vi "Offsets Widget.vi"(8 "error in (no error)":errorcluster) -> (0 "error out":errorcluster)   [LabVIEW 2013]
uses:
  Popups/Update Offset Actions.ctl
  lib/Data Access Objects/Metadata/Persistant DAO Actions.ctl
  lib/Data Access Objects/Metadata/DAO Actions.ctl
  lib/Global Data/Transactions/Dataset Source.ctl
  lib/Global Data/Transactions/Dataset Type.ctl
  lib/Apps/Yes No Button.ctl
  lib/Global Data/Transactions/Dataset Transaction Id.ctl
  lib/Data Access Objects/Metadata/DAO Actions with Remove.ctl
  lib/Launcher/Launcher Actions.ctl
  lib/Launcher/NoPanelAppTypes.ctl
  lib/Offsets/Offset Types.ctl
  Popups/Offset Message.ctl
  <vilib>/Utility/miscctls.llb/LVPointTypeDef.ctl
  lib/Data Display/External Sensor Name Offset & Value.ctl
  lib/Offsets Widget/Offset Widget Actions.ctl
  lib/MixedMode/Messages/MM Widget Parameter Changes.ctl
  lib/Apps/GUI Control.ctl
  lib/Data Access Objects/Sensors/Sensor List Class.lvclass
  Popups/Offset Table Component.ctl
  lib/Offsets Widget/Cartesian Or Actuator.ctl
panel:
  in  "HasBeenModified":bool
  in  "External Sensors Label":string[](array[string])
  in  "External Sensors Table":T1[](array[typedef])
  in  "Table 5":T2 {"Table Data 1" format="%^#_7e"}
  in  "Table 4":T2 {"Table Data 1" format="%^#_7e"}
  in  "Table 3":T2 {"Table Data 1" format="%^#_7e"}
  in  "Table 2":T2 {"Table Data 1" format="%^#_7e"}
  in  "Table 1":T2 {"Table Data 1" format="%^#_7e"}
  in  "Row Labels":string[](array[string])
  in  "Table 0":T2 {"Table Data 1" format="%^#_7e"}
  out "Default Data":dbl[][](array[numeric])
  out "Default Transactions":T3[](array[typedef])
  in  "Coordinate Space":T7 caption="Coord"
  in  "Cartesian Type":bool caption="Coord"
  in  "Offset Type":T8
  in  "Load":bool
  in  "Number Of Samples":i32
  in  "Sample Interval\n(milliseconds)":dbl
  in  "Offset Widget Actions":T9
  in  "Execute":bool
  in  "Cancel":bool
  in  "Ok":bool
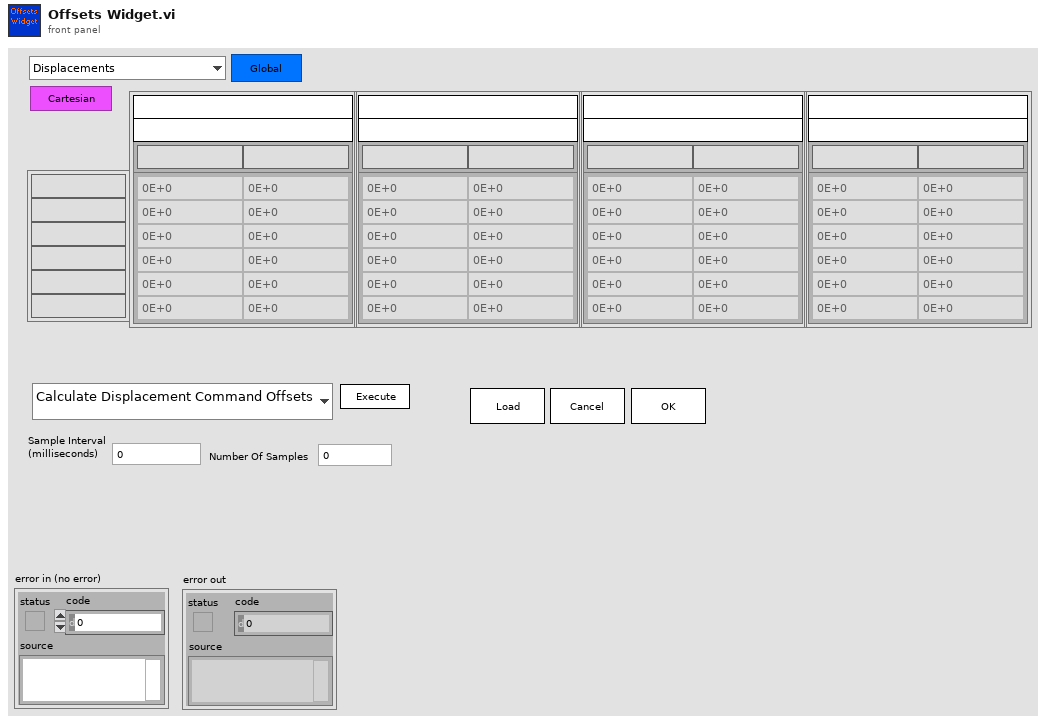
[diagram p1: front panel]
types:
  T1 = typedef "External Sensor Name Offset & Value.ctl" = cluster{"Name":string, "Offset":dbl, "Value 2":dbl}
  T2 = typedef "Offset Table Component.ctl" = cluster{"Table Data 1":dbl[][], "Offset or Current Label":string[], "DOF Label":string, "LBCB Label":string}
  T3 = typedef "Dataset Transaction Id.ctl" = cluster{"Dataset Source":T4, "Dataset Type":T5, "Hold":T6, "Volts":T6, "Tag":string}
  T4 = typedef "Dataset Source.ctl" = enum16{"Continuous", "Hold", "ED", "Volts", "Offsets", "Increments"}
  T5 = typedef "Dataset Type.ctl" = enum16{"LVDT", "Load Cell", "Actuator Command", "Servo Error", "Displacement Command", "Displacement", "Force"}
  T6 = typedef "Yes No Button.ctl" = bool
  T7 = typedef "Cartesian Or Actuator.ctl" = bool
  T8 = typedef "Offset Types.ctl" = enum16{"Displacements", "Forces", "External Sensors"}
  T9 = typedef "Offset Widget Actions.ctl" = enum16{"Calculate Displacement Command Offsets", "Calculate Displacement Offsets", "Calculate Force Offsets", "Calculate External Sensor Offsets"}
  T10 = typedef "GUI Control.ctl" = cluster{"Command":T11, "LBCB Number":enum16{"LBCB1", "LBCB2"}}
  T11 = typedef "MM Widget Parameter Changes.ctl" = enum16{"Start", "Stop All", "Control Enabled", "Control Disabled"}
  T12 = typedef "Offset Message.ctl" = cluster{"Update Offset Actions":T13, "Offset Type":T8, "Coordinate Space":bool, "Cartesian Type":bool}
  T13 = typedef "Update Offset Actions.ctl" = enum16{"Update Table", "Calculate Cartesian Offsets", "Redo Headers", "Has Been Modified", "Exit"}
  T14 = typedef "LVPointTypeDef.ctl" = cluster{"Horizontal":i16, "Vertical":i16}
  T15 = typedef "Persistant DAO Actions.ctl" = enum16{"Init", "Get", "Set", "Load", "Save"}
  T16 = typedef "DAO Actions.ctl" = enum16{"Init", "Get", "Set"}
  T17 = typedef "LVRectTypeDef.ctl" = cluster{"Left":i16, "Top":i16, "Right":i16, "Bottom":i16}
  T18 = typedef "App Parameters.ctl" = cluster{"Monitor Loop":T19, "Ramp Time":T19, "Log Loop":T19, "TCP to DAQ":T19, "Logging Directory":path, "Log File Size (MBytes)":i64, "Volt Logging Loop":T19, "2 LBCB Archiving Mode":bool, "Fake":bool}
  T19 = typedef "Timing Parameters.ctl" = cluster{"Interval":dbl, "Rate ":dbl}
  T20 = typedef "Number Of LBCBs.ctl" = enum16{"1", "2"}
  T21 = cluster{"Table Data 1":dbl[][], "Offset or Current Label":string[], "DOF Label":string, "LBCB Label":string}
  T22 = typedef "DAO Actions with Remove.ctl" = enum16{"Init", "Get", "Set", "Remove"}
  T23 = typedef "NoPanelAppTypes.ctl" = enum16{"NTCP Socket", "Data Archiving", "DAQ Link", "Control Loops", "Cmd Disp Diffs", "LBCB Data", "Limits", "Mixed Mode Widget", "Offsets", "Debug"}
  T24 = typedef "Launcher Actions.ctl" = enum16{"Launch", "Stop All", "Stop", "Kill", "Running?", "Init"}
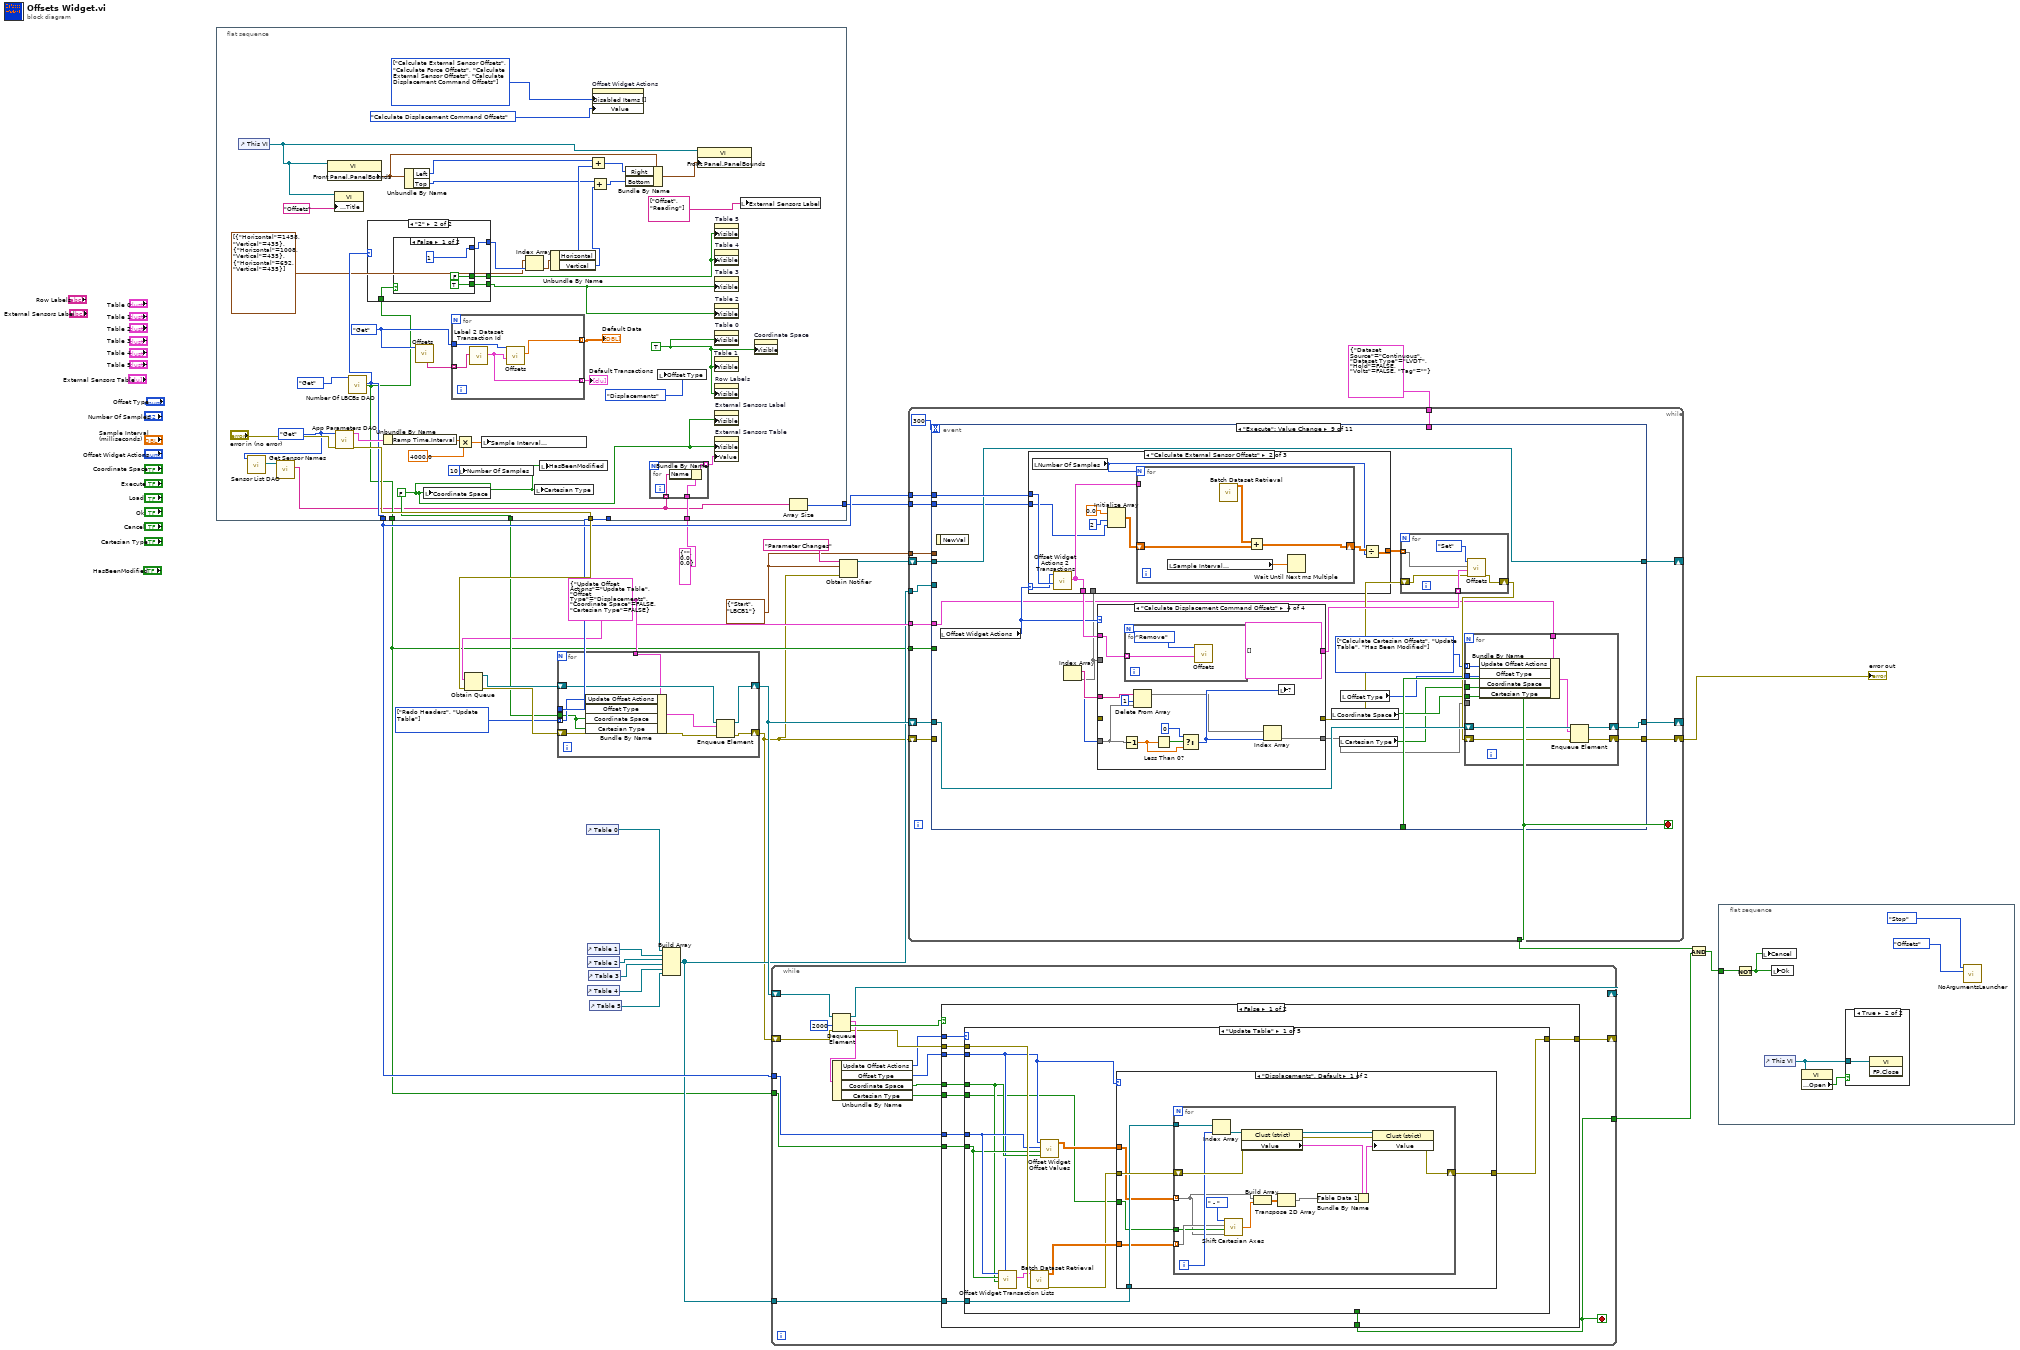
[diagram p0: block diagram]
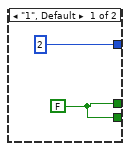
[diagram p2: hidden frame]
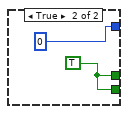
[diagram p3: hidden frame]
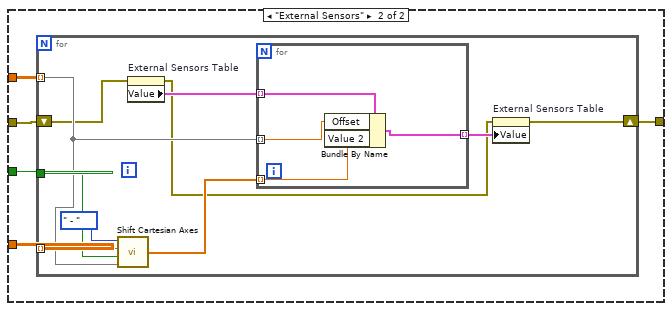
[diagram p5: hidden frame]
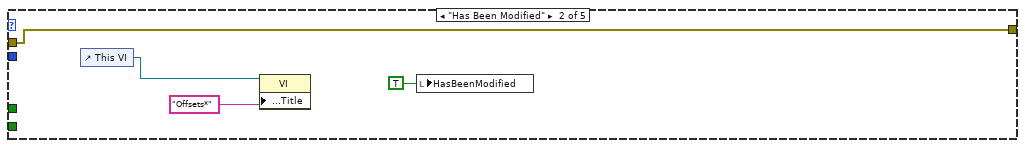
[diagram p6: hidden frame]
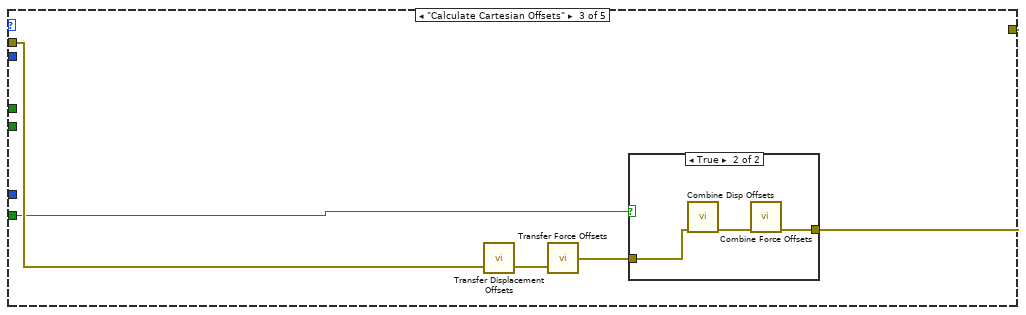
[diagram p7: hidden frame]
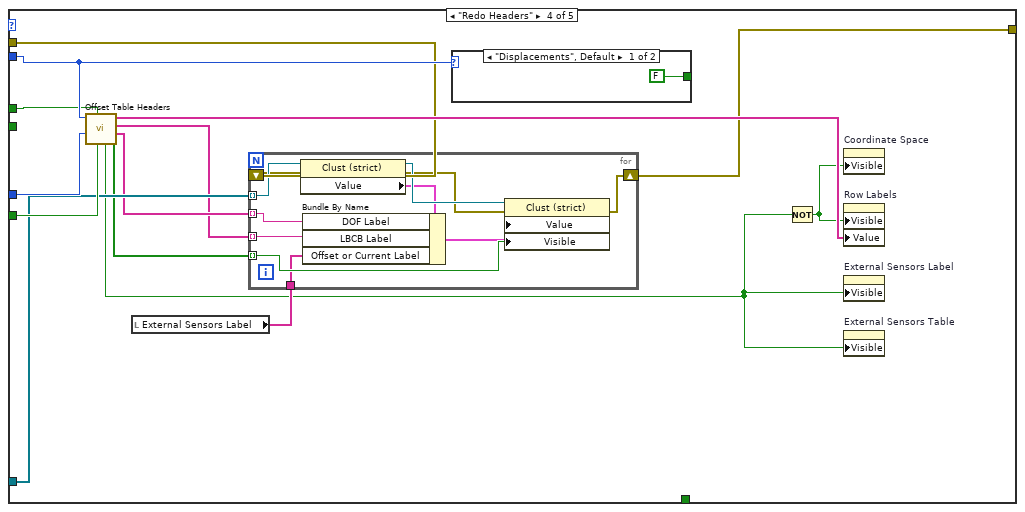
[diagram p9: hidden frame]
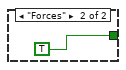
[diagram p10: hidden frame]
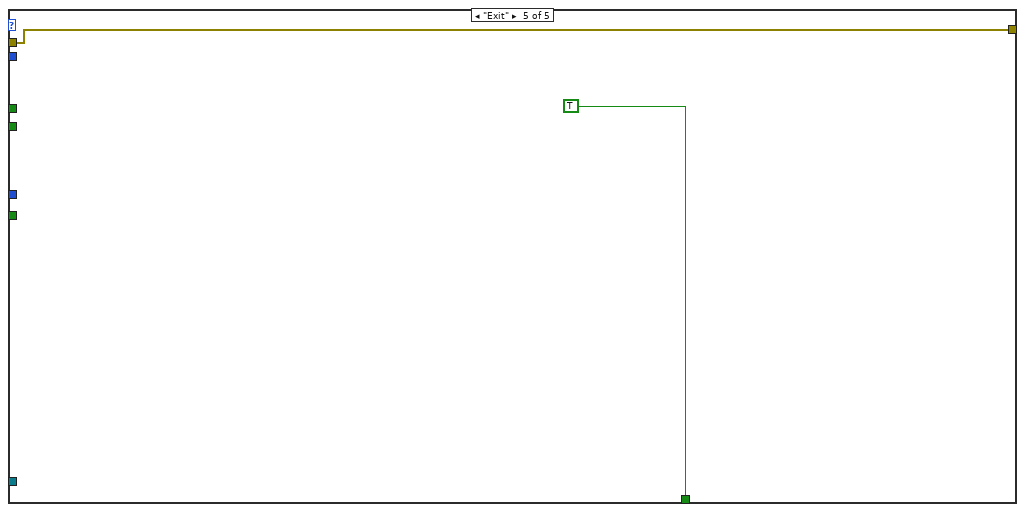
[diagram p11: hidden frame]
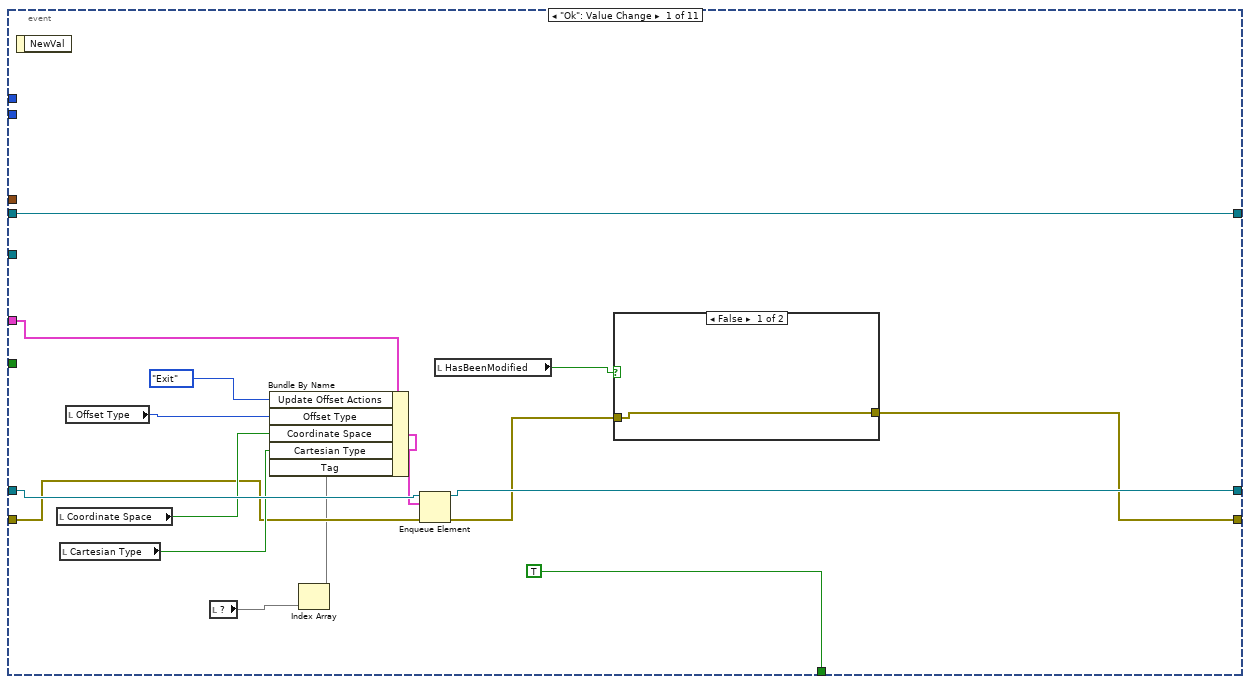
[diagram p13: hidden frame]
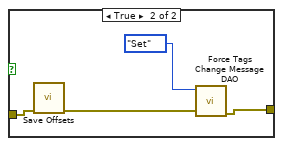
[diagram p14: hidden frame]
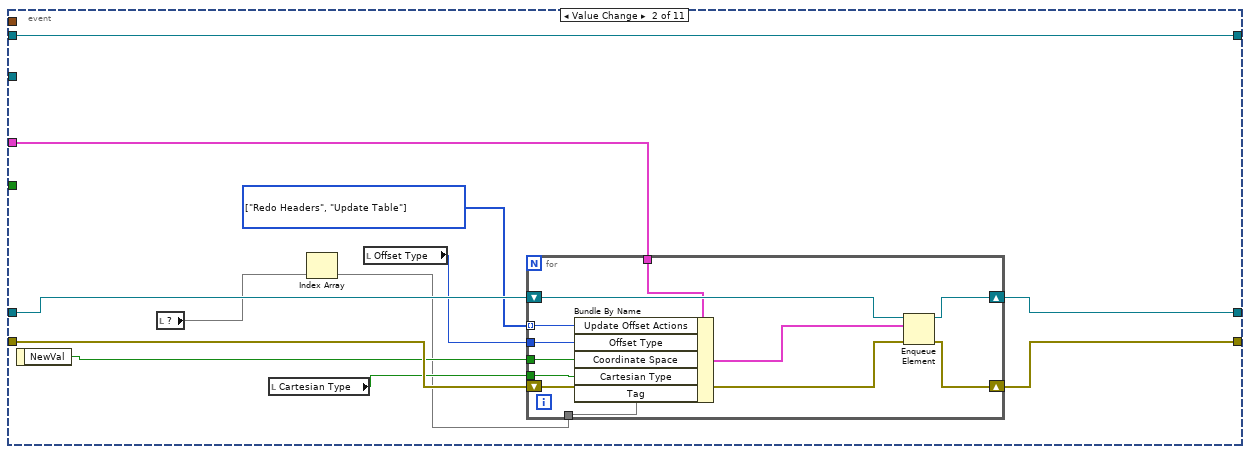
[diagram p15: hidden frame]
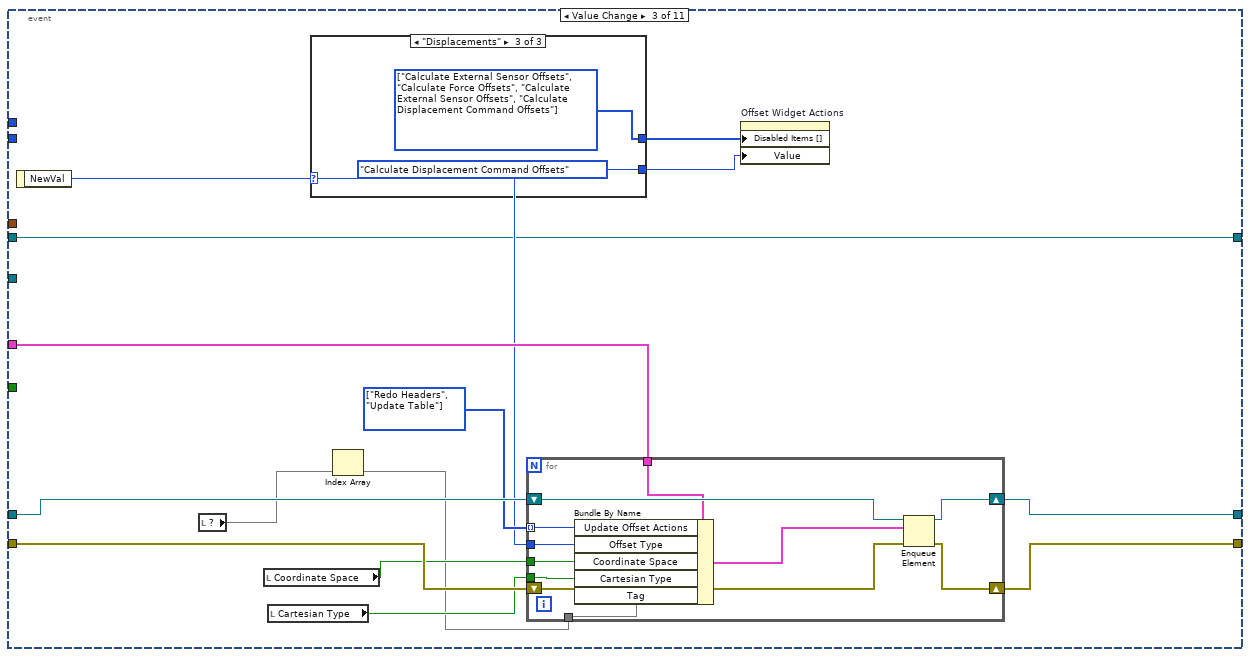
[diagram p16: hidden frame]
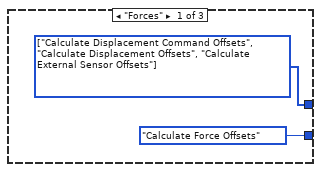
[diagram p17: hidden frame]
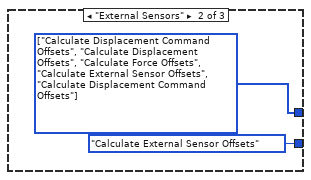
[diagram p18: hidden frame]
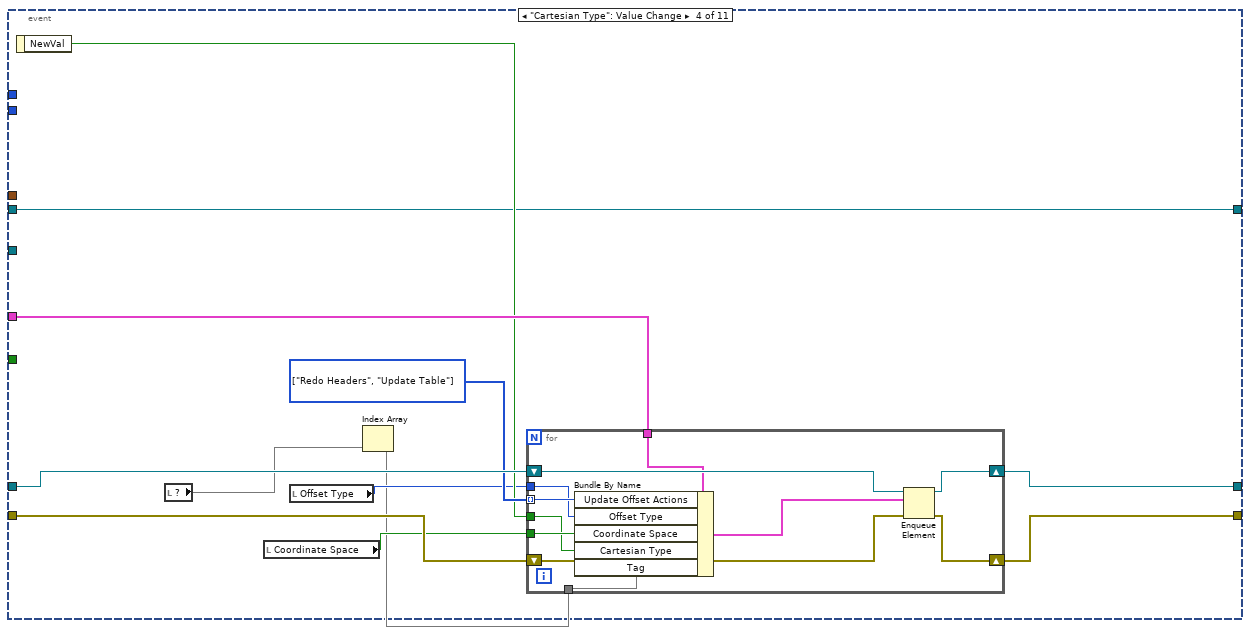
[diagram p19: hidden frame]
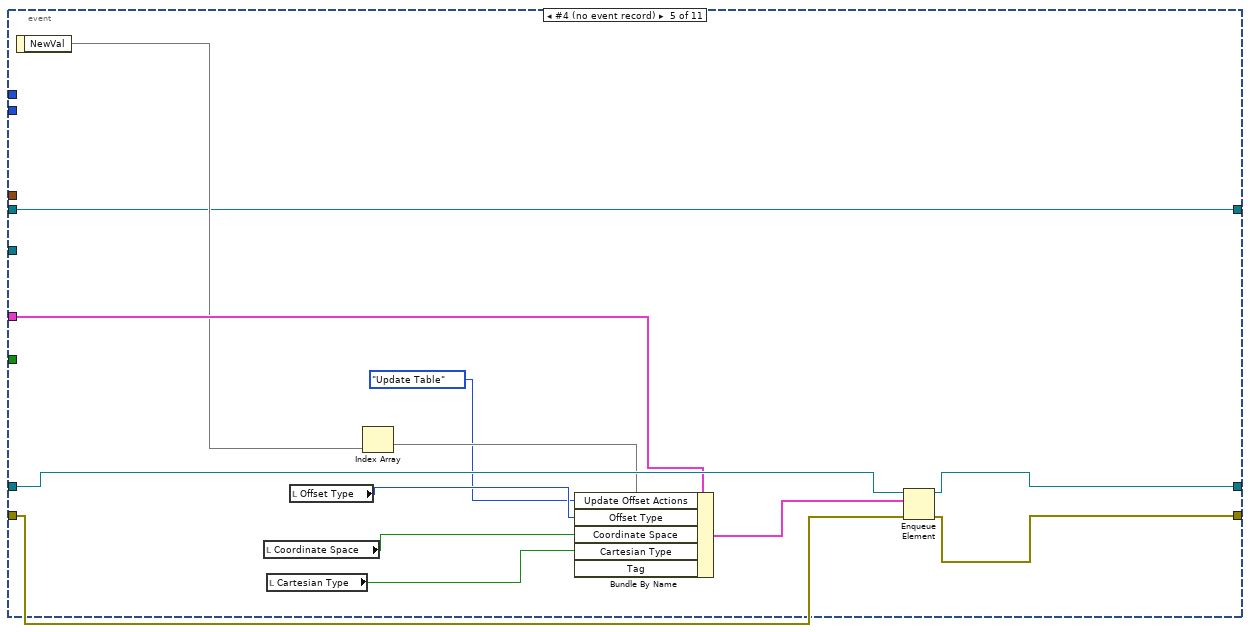
[diagram p20: hidden frame]
diagram:
  w2 = T10 {"Command"=enum."Start", "LBCB Number"=enum."LBCB1"} ("GUI Control")
  w16 = T12 {"Update Offset Actions"=enum."Update Table", "Offset Type"=enum."Displacements", "Coordinate Space"=FALSE, "Cartesian Type"=FALSE} ("Offset Message")
  w19 = T13[] [enum."Redo Headers", enum."Update Table"] items=["Update Table", "Calculate Cartesian Offsets", "Redo Headers", "Has Been Modified", "Exit"]
  n1 = flat-sequence {
    tunnel: [w59] -> w21
    tunnel: [w57] -> w20
    tunnel: [w56] -> w6
    tunnel: [w29] -> w18
    tunnel: [w35] -> w17
    tunnel: T1 {"Name"="", "Offset"=0.0, "Value 2"=0.0} ("External Sensor Name & Value") -> [w49]
    tunnel: [w33] -> w1
    frame #0 {
      w39 = T9[] [enum."Calculate External Sensor Offsets", enum."Calculate Force Offsets", enum."Calculate External Sensor Offsets", enum."Calculate Displacement Command Offsets"] items=["Calculate Displacement Command Offsets", "Calculate Displacement Offsets", "Calculate Force Offsets", "Calculate External Sensor Offsets"] ("Disabled Items []")
      w34 = TRUE ("Visible")
      w35 = FALSE ("Coordinate Space")
      w60 = DAO_Actions."Get" ("DAO Actions")
      w31 = Persistant_DAO_Actions."Get" ("Actions")
      n2 = control-ref of="This VI"() -> (w37:refnum<vi>)
      n3 = call "Sensor List DAO.vi"("Actions"=w31) -> ("Sensor List Out"=w32:refnum<class "Sensor List Class.lvclass">)  [unwired: 8 in, 2 out]
      n4 = call "Get Sensor Names.vi"("Sensor List Class in"=w32) -> ("Names"=w30:string[])  [unwired: 8 in, 2 out]
      n5 = property class="VI"(reference=w37) -> ("Front Panel.PanelBounds"=w44:T17)  [unwired: 1 in, 2 out]
      n6 = property class="VI"(reference=w37, "Front Panel.Title"="Offsets" ("Front Panel Window:Title")) -> ()  [unwired: 1 in, 2 out]
      n7 = call "App Parameters DAO.vi"("error in (no error)"="error in (no error)", "Actions"=w31) -> ("error out"=w59:errorcluster, "Application Timing and Logging Out"=w66:T18)  [unwired: 2 in, 6 out]
      n8 = call "Number Of LBCBs DAO.vi"("Actions"=Persistant_DAO_Actions."Get") -> ("Number of\nLBCBs Out"=w57:T20, "Rigid Connection Out"=w56:bool)  [unwired: 13 in, 4 out]
      n9 = case shown="\"2\"" w57 {
        tunnel: w56 -> [_ w79]
        tunnel: [2 w78] -> w55
        tunnel: [w74 w77] -> w52
        tunnel: [w74 w76] -> w51
        frame "1", Default {
          w74 = FALSE
        }
        frame "2" {
          n10 = case shown="False" w79 {
            tunnel: [1 ("f") 0] -> w78
            tunnel: [FALSE w83] -> w77
            tunnel: [TRUE w83] -> w76
            frame False {
            }
            frame True {
              w83 = TRUE
            }
          }
        }
      }
      n11 = Unbundle By Name(w66) -> ("Ramp Time.Interval"=w67:dbl)
      n12 = Unbundle By Name(w44) -> ("Left"=w48:i16, "Top"=w46:i16)
      n13 = call "Offsets.vi"("DAO Actions"=w60) -> ("Labels"=w64:string[])  [unwired: 8 in, 2 out]
      n14 = local write "Coordinate Space"(w35) -> ()
      n15 = for {
        tunnel: w64 -> [w88] mode=indexing
        tunnel: w60 -> [w87]
        tunnel: [w86] -> w63 mode=indexing
        tunnel: [w85] -> w62 mode=indexing
        n16 = call "Label 2 Dataset Transaction Id.vi"("Label"=w88) -> ("Dataset Trans Id"=w86:T3)  [unwired: 10 in]
        n17 = call "Offsets.vi"("Dataset Trans Id"=w86, "DAO Actions"=w87) -> ("Data Out"=w85:dbl[])  [unwired: 7 in, 2 out]
      }
      "Default Transactions" <- w63
      "Default Data" <- w62
      n18 = Multiply(x=w67, y=4000.0) -> (x*y=w69:dbl)
      n19 = local write "Number Of Samples"(10 ("Number Of Samples")) -> ()
      n20 = local write "Sample Interval\n(milliseconds)"(w69) -> ()
      n21 = Index Array(array=T14[] [{"Horizontal"=1458, "Vertical"=435}, {"Horizontal"=1008, "Vertical"=435}, {"Horizontal"=692, "Vertical"=435}], index=w55) -> (element=w53:T14)
      n22 = local write "Cartesian Type"(w35) -> ()
      n23 = local write "HasBeenModified"(w35) -> ()
      n24 = Unbundle By Name(w53) -> ("Horizontal"=w47:i16, "Vertical"=w45:i16)
      n25 = Add(x=w48, y=w47) -> (x+y=w42:i16)
      n26 = Add(x=w46, y=w45) -> (x+y=w41:i16)
      n27 = property on="Offset Widget Actions" class="Enum (strict)"("Disabled Items []"=w39, "Value"=Offset_Widget_Actions."Calculate Displacement Command Offsets" ("Offset Widget Actions")) -> ()  [unwired: 2 in, 2 out]
      n28 = Bundle By Name(cluster=w44, "Right"=w42, "Bottom"=w41) -> (w43:T17)
      n29 = for {
        tunnel: [w73] -> w50 mode=indexing
        tunnel: w49 -> [w72]
        tunnel: w30 -> [w71] mode=indexing
        n30 = Bundle By Name(cluster=w72, "Name"=w71) -> (w73:T1)
      }
      n31 = local write "Offset Type"(Offset_Types."Displacements" ("Offset Type")) -> ()
      n32 = property class="VI"(reference=w37, "Front Panel.PanelBounds"=w43) -> ()  [unwired: 1 in, 2 out]
      n33 = property on="Table 5" class="Clust (strict)"("Visible"=w52) -> ()  [unwired: 2 in, 2 out]
      n34 = property on="Table 4" class="Clust (strict)"("Visible"=w52) -> ()  [unwired: 2 in, 2 out]
      n35 = property on="Table 3" class="Clust (strict)"("Visible"=w51) -> ()  [unwired: 2 in, 2 out]
      n36 = property on="Table 2" class="Clust (strict)"("Visible"=w51) -> ()  [unwired: 2 in, 2 out]
      n37 = property on="Table 0" class="Clust (strict)"("Visible"=w34) -> ()  [unwired: 2 in, 2 out]
      n38 = property on="Table 1" class="Clust (strict)"("Visible"=w34) -> ()  [unwired: 2 in, 2 out]
      n39 = property on="Row Labels" class="Arr (strict)"("Visible"=w34) -> ()  [unwired: 2 in, 2 out]
      n40 = property on="External Sensors Label" class="Arr (strict)"("Visible"=w35) -> ()  [unwired: 2 in, 2 out]
      n41 = property on="External Sensors Table" class="Arr (strict)"("Visible"=w35, "Value"=w50) -> ()  [unwired: 2 in, 2 out]
      n42 = local write "External Sensors Label"(string[] ["Offset", "Reading"] ("External Sensors Label")) -> ()
      n43 = property on="Coordinate Space" class="Bool (strict)"("Visible"=w34) -> ()  [unwired: 2 in, 2 out]
      n44 = Array Size(array=w30) -> (size(s)=w33:i32)
    }
  }
  n45 = Obtain Queue(element data type=w16, error in (no error)=w21) -> (queue out=w27:refnum<queue>, error out=w28:errorcluster)  [unwired: 3 in, 1 out]
  n46 = for {
    tunnel: w19 -> [w93] mode=indexing
    shift-right: [w94] -> w26
    shift-left: w27 -> [w95]
    shift-right: [w92] -> w3
    shift-left: w28 -> [w96]
    tunnel: w16 -> [w90]
    tunnel: w18 -> [_]
    tunnel: w17 -> [w89]
    n47 = Bundle By Name(cluster=w90, "Update Offset Actions"=w93, "Coordinate Space"=w89, "Cartesian Type"=w89) -> (w91:T12)  [unwired: 1 in]
    n48 = Enqueue Element(queue=w95, element=w91, error in (no error)=w96) -> (queue out=w94:refnum<queue>, error out=w92:errorcluster)  [unwired: 1 in, 1 out]
  }
  n49 = control-ref of="Table 0"() -> (w15:refnum<vi>)
  n50 = control-ref of="Table 1"() -> (w14:refnum<vi>)
  n51 = control-ref of="Table 2"() -> (w13:refnum<vi>)
  n52 = control-ref of="Table 4"() -> (w11:refnum<vi>)
  n53 = control-ref of="Table 3"() -> (w12:refnum<vi>)
  n54 = control-ref of="Table 5"() -> (w10:refnum<vi>)
  n55 = Build Array(w15, w14, w13, w12, w11, w10) -> (w8:refnum<vi>[])
  n56 = while {
    shift-right: [w109] -> _
    shift-left: w26 -> [w111]
    shift-right: [w105] -> _
    shift-left: w3 -> [w110]
    tunnel: [w104] -> w23
    tunnel: w20 -> [w103]
    tunnel: w6 -> [w102]
    tunnel: w8 -> [w98]
    stop <- w104 stop-if-true
    n57 = Dequeue Element(queue=w111, timeout in ms (-1)=2000, error in (no error)=w110) -> (queue out=w109:refnum<queue>, element=w107:T12, timed out?=w108:bool, error out=w106:errorcluster)
    n58 = Unbundle By Name(w107) -> ("Update Offset Actions"=w101:T13, "Offset Type"=w100:T8, "Coordinate Space"=w99:bool, "Cartesian Type"=w97:bool)
    n59 = case shown="False" w108 {
      tunnel: w101 -> [w122 _]
      tunnel: w106 -> [w121 w219]
      tunnel: [w120 w219] -> w105
      tunnel: [w119 _] -> w104
      tunnel: w100 -> [w118 _]
      tunnel: w103 -> [w117 _]
      tunnel: w102 -> [w116 _]
      tunnel: w99 -> [w115 _]
      tunnel: w98 -> [w114 _]
      tunnel: w97 -> [w113 _]
      frame False {
        n60 = case shown="\"Update Table\"" w122 {
          tunnel: w121 -> [w134 w176 w181 w192 w217]
          tunnel: [w125 w176 w183 w193 w217] -> w120
          tunnel: [_ _ _ _ TRUE] -> w119
          tunnel: w118 -> [w124 _ _ w202 _]
          tunnel: w117 -> [w131 _ _ w201 _]
          tunnel: w116 -> [w130 _ w180 w199 _]
          tunnel: w115 -> [w129 _ _ w200 _]
          tunnel: w114 -> [w127 _ _ w197 _]
          tunnel: w113 -> [w123 _ _ _ _]
          frame "Update Table" {
            n61 = call "Offset Widget Transaction Lists.vi"("Offset Type"=w124, "Coordinate Space"=w129, "Rigid Connection"=w130, "Number of\nLBCBs"=w131) -> ("Transactions"=w128:T3[])  [unwired: 6 in, 1 out]
            n62 = call "Batch Dataset Retrieval.vi"("error in"=w134, "Transactions"=w128) -> ("error out"=w126:errorcluster, "Data"=w133:dbl[][])  [unwired: 8 in]
            n63 = call "Offset Widget Offset Values.vi"("Coordinate Space"=w129, "Rigid Connection In"=w130, "Number of\nLBCBs"=w131, "Offset Type"=w124) -> ("Offsets"=w132:dbl[][])  [unwired: 7 in]
            n64 = case shown="\"Displacements\", Default" w124 {
              tunnel: w133 -> [w137 w161]
              tunnel: w132 -> [w136 w160]
              tunnel: w123 -> [w135 w159]
              tunnel: w127 -> [w138 _]
              tunnel: w126 -> [w140 w158]
              tunnel: [w139 w157] -> w125
              frame "Displacements", Default {
                n65 = for {
                  shift-right: [w154] -> w139
                  shift-left: w140 -> [w156]
                  tunnel: w138 -> [w153]
                  tunnel: w137 -> [w147] mode=indexing
                  tunnel: w136 -> [w145] mode=indexing
                  tunnel: w135 -> [w146]
                  i -> [w152]
                  n66 = Index Array(array=w153, index=w152) -> (element=w151:refnum<vi>)
                  n67 = call "Shift Cartesian Axes.vi"("Coordinate Offset"=w145, "Coordinate Switch"=w146, "Coordinate Input"=w147, "Direction"=enum16{" +", " - "}." - ") -> ("Coordinate Output"=w144:dbl[])
                  n68 = property class="Clust (strict)"(reference=w151, error in=w156) -> (reference out=w150:refnum<vi>, error out=w155:errorcluster, "Value"=w149:T21)
                  n69 = Build Array(w145, w144) -> (w143:dbl[][])
                  n70 = Transpose 2D Array(2D array=w143) -> (transposed array=w142:dbl[][])
                  n71 = Bundle By Name(cluster=w149, "Table Data 1"=w142) -> (w141:T21)
                  n72 = property class="Clust (strict)"(reference=w150, error in=w155, "Value"=w141) -> (error out=w154:errorcluster)  [unwired: 1 out]
                }
              }
              frame "External Sensors" {
                n73 = for {
                  tunnel: w161 -> [w171] mode=indexing
                  tunnel: w159 -> [w170]
                  tunnel: w160 -> [w167] mode=indexing
                  shift-right: [w164] -> w157
                  shift-left: w158 -> [w163]
                  n74 = call "Shift Cartesian Axes.vi"("Coordinate Offset"=w167, "Coordinate Switch"=w170, "Coordinate Input"=w171, "Direction"=enum16{" +", " - "}." - ") -> ("Coordinate Output"=w166:dbl[])
                  n75 = property on="External Sensors Table" class="Arr (strict)"(error in=w163) -> (error out=w162:errorcluster, "Value"=w168:T1[])  [unwired: 1 in, 1 out]
                  n76 = for {
                    tunnel: w168 -> [w175] mode=indexing
                    tunnel: w167 -> [w174] mode=indexing
                    tunnel: w166 -> [w173] mode=indexing
                    tunnel: [w172] -> w165 mode=indexing
                    n77 = Bundle By Name(cluster=w175, "Offset"=w174, "Value 2"=w173) -> (w172:T1)
                  }
                  n78 = property on="External Sensors Table" class="Arr (strict)"(error in=w162, "Value"=w165) -> (error out=w164:errorcluster)  [unwired: 1 in, 1 out]
                }
              }
            }
          }
          frame "Has Been Modified" {
            n79 = control-ref of="This VI"() -> (w179:refnum<vi>)
            n80 = property class="VI"(reference=w179, "Front Panel.Title"="Offsets*" ("Front Panel Window:Title")) -> ()  [unwired: 1 in, 2 out]
            n81 = local write "HasBeenModified"(TRUE ("HasBeenModified")) -> ()
          }
          frame "Calculate Cartesian Offsets" {
            n82 = call "Transfer Displacement Offsets.vi"("error in"=w181) -> ("error out"=w182:errorcluster)  [unwired: 2 in]
            n83 = call "Transfer Force Offsets.vi"("error in"=w182) -> ("error out"=w184:errorcluster)  [unwired: 1 in]
            n84 = case shown="True" w180 {
              tunnel: w184 -> [w185 w188]
              tunnel: [w185 w186] -> w183
              frame False {
              }
              frame True {
                n85 = call "Combine Disp Offsets.vi"("error in (no error)"=w188) -> ("error out"=w187:errorcluster)  [unwired: 10 in]
                n86 = call "Combine Force Offsets.vi"("error in (no error)"=w187) -> ("error out"=w186:errorcluster)  [unwired: 10 in]
              }
            }
          }
          frame "Redo Headers" {
            n87 = call "Offset Table Headers.vi"("Rigid Connection"=w199, "Coordinate Space"=w200, "Number of\nLBCBs"=w201, "Offset Type"=w202) -> ("Visible"=w194:bool[], "Column DOF Headers"=w196:string[], "Column LBCB Headers"=w195:string[], "Row Headers"=w198:string[], "Ext Visible"=w190:bool)  [unwired: 3 in]
            n88 = local read "External Sensors Label"() -> (w191:string[])
            n89 = for {
              tunnel: w197 -> [w209] mode=indexing
              tunnel: w196 -> [w212] mode=indexing
              tunnel: w195 -> [w213] mode=indexing
              tunnel: w194 -> [w214] mode=indexing
              shift-right: [w210] -> w193
              shift-left: w192 -> [w207]
              tunnel: w191 -> [w204]
              n90 = property class="Clust (strict)"(reference=w209, error in=w207) -> (reference out=w208:refnum<vi>, error out=w206:errorcluster, "Value"=w205:T21)
              n91 = Bundle By Name(cluster=w205, "DOF Label"=w212, "LBCB Label"=w213, "Offset or Current Label"=w204) -> (w211:T21)
              n92 = property class="Clust (strict)"(reference=w208, error in=w206, "Value"=w211, "Visible"=w214) -> (error out=w210:errorcluster)  [unwired: 1 out]
            }
            n93 = case shown="\"Displacements\", Default" w202 {
              tunnel: [FALSE TRUE] -> w203
              frame "Displacements", Default {
              }
              frame "Forces" {
              }
            }
            n94 = Not(x=w190) -> (.not. x?=w189:bool)
            n95 = property on="Coordinate Space" class="Bool (strict)"("Visible"=w189) -> ()  [unwired: 2 in, 2 out]
            n96 = property on="Row Labels" class="Arr (strict)"("Visible"=w189, "Value"=w198) -> ()  [unwired: 2 in, 2 out]
            n97 = property on="External Sensors Label" class="Arr (strict)"("Visible"=w190) -> ()  [unwired: 2 in, 2 out]
            n98 = property on="External Sensors Table" class="Arr (strict)"("Visible"=w190) -> ()  [unwired: 2 in, 2 out]
          }
          frame "Exit" {
          }
        }
      }
      frame True {
      }
    }
  }
  n99 = Obtain Notifier(name (unnamed)="Parameter Changes", notification data type=w2, error in (no error)=w3) -> (notifier out=w4:refnum<notifier>)  [unwired: 1 in, 2 out]
  n100 = while {
    shift-right: [w232] -> _
    shift-left: w26 -> [w234]
    shift-right: [w231] -> w25
    shift-left: w3 -> [w233]
    tunnel: [w229] -> w24
    tunnel: w20 -> [w228]
    tunnel: w16 -> [w227]
    tunnel: w8 -> [w226]
    tunnel: T3 {"Dataset Source"=enum."Continuous", "Dataset Type"=enum."LVDT", "Hold"=FALSE, "Volts"=FALSE, "Tag"=""} ("Dataset Trans Id") -> [w225]
    tunnel: w6 -> [w224]
    tunnel: w2 -> [w222]
    shift-right: [w221] -> _
    shift-left: w4 -> [w223]
    tunnel: w1 -> [w220]
    stop <- w229 stop-if-true
    n101 = event shown="[8] \"Execute\": Value Change" {
      selector: _ -> [_ _ _ _ _ _ _ _ _ _ _]
      dyn-events: _ -> [_ _ _ _ _ _ _ _ _ _ _]
      timeout: 300 -> [_ _ _ _ _ _ _ _ _ _ _]
      tunnel: [TRUE _ _ _ _ _ TRUE TRUE _ _ _] -> w229
      tunnel: w234 -> [w250 w269 w295 w325 w350 w356 w403 w420 w444 w541 w635]
      tunnel: w233 -> [w240 w268 w294 w324 w349 w359 w400 w417 w434 w553 w632]
      tunnel: [w249 w266 w292 w322 w347 w355 w402 w419 w442 w542 w634] -> w232
      tunnel: [w238 w267 w293 w323 w348 w352 w401 w418 w443 w543 w633] -> w231
      tunnel: w228 -> [_ _ _ _ _ _ _ _ w441 w547 _]
      tunnel: w227 -> [w247 w264 w290 w320 w346 w354 w396 w413 w430 w538 w630]
      tunnel: w226 -> [_ _ _ _ _ _ _ _ _ w551 _]
      tunnel: w225 -> [_ _ _ _ _ _ _ _ _ w548 _]
      tunnel: w224 -> [_ _ _ _ _ _ _ _ _ w546 _]
      tunnel: w223 -> [w235 w257 w281 w313 w337 w357 w388 w405 w424 w533 w638]
      tunnel: w222 -> [_ _ _ _ _ _ _ _ _ _ _]
      tunnel: [w235 w257 w281 w313 w337 w357 w388 w405 w424 w533 w638] -> w221
      tunnel: w220 -> [_ _ _ _ _ _ _ _ w422 _ _]
      event "Ok": Value Change {
        n102 = event-data() -> ()  [unwired: 2 out]
        n103 = local read "Coordinate Space"() -> (w244:T7)
        n104 = local read "Cartesian Type"() -> (w243:bool)
        n105 = local read "Offset Type"() -> (w245:T8)
        n106 = local read item#-1() -> (w241)
        n107 = Index Array(index=w241) -> (array=w242:string[], element=w236)
        n108 = Bundle By Name(cluster=w247, "Update Offset Actions"=Update_Offset_Actions."Exit" ("notification"), "Offset Type"=w245, "Coordinate Space"=w244, "Cartesian Type"=w243, "Tag"=w236) -> (w248:T12)
        n109 = Enqueue Element(queue=w250, element=w248, error in (no error)=w240) -> (queue out=w249:refnum<queue>, error out=w239:errorcluster)  [unwired: 1 in, 1 out]
        n110 = local read "HasBeenModified"() -> (w237:bool)
        n111 = case shown="False" w237 {
          tunnel: w239 -> [w252 w256]
          tunnel: [w252 w253] -> w238
          frame False {
          }
          frame True {
            n112 = call "Save Offsets.vi"("error in (no error)"=w256) -> ("error out"=w255:errorcluster)  [unwired: 10 out]
            n113 = call "Force Tags Change Message DAO.vi"("error in (no error)"=w255, "DAO Actions"=DAO_Actions."Set") -> ("error out"=w253:errorcluster)  [unwired: 7 in, 2 out]
          }
        }
      }
      event Value Change {
        w265 = T13[] [enum."Redo Headers", enum."Update Table"] items=["Update Table", "Calculate Cartesian Offsets", "Redo Headers", "Has Been Modified", "Exit"]
        n114 = event-data() -> ("NewVal"=w263:T7)  [unwired: 1 out]
        n115 = local read item#-1() -> (w260)
        n116 = local read "Cartesian Type"() -> (w261:bool)
        n117 = Index Array(index=w260) -> (array=w259:string[], element=w258)
        n118 = local read "Offset Type"() -> (w262:T8)
        n119 = for {
          tunnel: w265 -> [w276] mode=indexing
          shift-right: [w277] -> w266
          shift-left: w269 -> [w280]
          shift-right: [w278] -> w267
          shift-left: w268 -> [w279]
          tunnel: w264 -> [w274]
          tunnel: w263 -> [w273]
          tunnel: w262 -> [w272]
          tunnel: w261 -> [w271]
          tunnel: w258 -> [w270]
          n120 = Bundle By Name(cluster=w274, "Update Offset Actions"=w276, "Offset Type"=w272, "Coordinate Space"=w273, "Cartesian Type"=w271, "Tag"=w270) -> (w275:T12)
          n121 = Enqueue Element(queue=w280, element=w275, error in (no error)=w279) -> (queue out=w277:refnum<queue>, error out=w278:errorcluster)  [unwired: 1 in, 1 out]
        }
      }
      event Value Change {
        w291 = T13[] [enum."Redo Headers", enum."Update Table"] items=["Update Table", "Calculate Cartesian Offsets", "Redo Headers", "Has Been Modified", "Exit"]
        n122 = event-data() -> ("NewVal"=w287:T8)  [unwired: 1 out]
        n123 = local read item#-1() -> (w284)
        n124 = local read "Coordinate Space"() -> (w289:T7)
        n125 = local read "Cartesian Type"() -> (w288:bool)
        n126 = case shown="\"Displacements\"" w287 {
          tunnel: [w297 w299 w301] -> w286
          tunnel: [Offset_Widget_Actions."Calculate Force Offsets" ("Offset Widget Actions") Offset_Widget_Actions."Calculate External Sensor Offsets" ("Offset Widget Actions") Offset_Widget_Actions."Calculate Displacement Command Offsets" ("Offset Widget Actions")] -> w285
          frame "Forces" {
            w297 = T9[] [enum."Calculate Displacement Command Offsets", enum."Calculate Displacement Offsets", enum."Calculate External Sensor Offsets"] items=["Calculate Displacement Command Offsets", "Calculate Displacement Offsets", "Calculate Force Offsets", "Calculate External Sensor Offsets"] ("Disabled Items []")
          }
          frame "External Sensors" {
            w299 = T9[] [enum."Calculate Displacement Command Offsets", enum."Calculate Displacement Offsets", enum."Calculate Force Offsets", enum."Calculate External Sensor Offsets", enum."Calculate Displacement Command Offsets"] items=["Calculate Displacement Command Offsets", "Calculate Displacement Offsets", "Calculate Force Offsets", "Calculate External Sensor Offsets"] ("Disabled Items []")
          }
          frame "Displacements" {
            w301 = T9[] [enum."Calculate External Sensor Offsets", enum."Calculate Force Offsets", enum."Calculate External Sensor Offsets", enum."Calculate Displacement Command Offsets"] items=["Calculate Displacement Command Offsets", "Calculate Displacement Offsets", "Calculate Force Offsets", "Calculate External Sensor Offsets"] ("Disabled Items []")
          }
        }
        n127 = Index Array(index=w284) -> (array=w283:string[], element=w282)
        n128 = for {
          tunnel: w291 -> [w308] mode=indexing
          shift-right: [w309] -> w292
          shift-left: w295 -> [w312]
          shift-right: [w310] -> w293
          shift-left: w294 -> [w311]
          tunnel: w290 -> [w306]
          tunnel: w289 -> [w305]
          tunnel: w287 -> [w304]
          tunnel: w288 -> [w303]
          tunnel: w282 -> [w302]
          n129 = Bundle By Name(cluster=w306, "Update Offset Actions"=w308, "Offset Type"=w304, "Coordinate Space"=w305, "Cartesian Type"=w303, "Tag"=w302) -> (w307:T12)
          n130 = Enqueue Element(queue=w312, element=w307, error in (no error)=w311) -> (queue out=w309:refnum<queue>, error out=w310:errorcluster)  [unwired: 1 in, 1 out]
        }
        n131 = property on="Offset Widget Actions" class="Enum (strict)"("Disabled Items []"=w286, "Value"=w285) -> ()  [unwired: 2 in, 2 out]
      }
      event "Cartesian Type": Value Change {
        w321 = T13[] [enum."Redo Headers", enum."Update Table"] items=["Update Table", "Calculate Cartesian Offsets", "Redo Headers", "Has Been Modified", "Exit"]
        n132 = event-data() -> ("NewVal"=w318:bool)  [unwired: 1 out]
        n133 = local read item#-1() -> (w316)
        n134 = local read "Coordinate Space"() -> (w319:T7)
        n135 = local read "Offset Type"() -> (w317:T8)
        n136 = Index Array(index=w316) -> (array=w315:string[], element=w314)
        n137 = for {
          tunnel: w321 -> [w332] mode=indexing
          shift-right: [w333] -> w322
          shift-left: w325 -> [w336]
          shift-right: [w334] -> w323
          shift-left: w324 -> [w335]
          tunnel: w320 -> [w330]
          tunnel: w319 -> [w329]
          tunnel: w318 -> [w328]
          tunnel: w317 -> [w327]
          tunnel: w314 -> [w326]
          n138 = Bundle By Name(cluster=w330, "Update Offset Actions"=w332, "Offset Type"=w327, "Coordinate Space"=w329, "Cartesian Type"=w328, "Tag"=w326) -> (w331:T12)
          n139 = Enqueue Element(queue=w336, element=w331, error in (no error)=w335) -> (queue out=w333:refnum<queue>, error out=w334:errorcluster)  [unwired: 1 in, 1 out]
        }
      }
      event #4 (no event record) {
        n140 = event-data() -> ("NewVal"=w341)  [unwired: 1 out]
        n141 = local read "Coordinate Space"() -> (w345:T7)
        n142 = local read "Cartesian Type"() -> (w340:bool)
        n143 = local read "Offset Type"() -> (w344:T8)
        n144 = Index Array(index=w341) -> (array=w343:string[], element=w342)
        n145 = Bundle By Name(cluster=w346, "Update Offset Actions"=Update_Offset_Actions."Update Table" ("element"), "Offset Type"=w344, "Coordinate Space"=w345, "Cartesian Type"=w340, "Tag"=w342) -> (w338:T12)
        n146 = Enqueue Element(queue=w350, element=w338, error in (no error)=w349) -> (queue out=w347:refnum<queue>, error out=w348:errorcluster)  [unwired: 1 in, 1 out]
      }
      event "Load": Mouse Down? {
        n147 = event-data() -> ()  [unwired: 3 out]
        n148 = local read "Offset Type"() -> (w353:T8)
        n149 = call "Load Offsets.vi"("error in (no error)"=w359) -> ("error out"=w351:errorcluster)  [unwired: 10 in]
        n150 = case shown="No Error" w351 {
          selector: w351 -> [w370 w386]
          tunnel: w356 -> [w373 w387]
          tunnel: [w361 w387] -> w355
          tunnel: w354 -> [w372 _]
          tunnel: w353 -> [w371 _]
          tunnel: [w360 w385] -> w352
          frame No Error {
            w362 = T13[] [enum."Calculate Cartesian Offsets", enum."Update Table"] items=["Update Table", "Calculate Cartesian Offsets", "Redo Headers", "Has Been Modified", "Exit"]
            w363 = u16 0 items=["<None>"] ("Force Offset Tag")
            n151 = local read "Coordinate Space"() -> (w369:T7)
            n152 = local read "Cartesian Type"() -> (w368:bool)
            n153 = call "Force Tags Change Message DAO.vi"("error in (no error)"=w370, "DAO Actions"=DAO_Actions."Get") -> ("error out"=w366:errorcluster, "Force Tags"=w365:string[])  [unwired: 7 in, 1 out]
            n154 = Index Array(array=w365, index=w363) -> (element=w367:string)
            n155 = local write item#-1(w363) -> ()
            n156 = for {
              tunnel: w372 -> [w379]
              tunnel: w371 -> [w378]
              tunnel: w369 -> [w377]
              tunnel: w368 -> [w376]
              tunnel: w367 -> [w375]
              tunnel: w362 -> [w374] mode=indexing
              shift-right: [w382] -> w361
              shift-left: w373 -> [w383]
              shift-right: [w381] -> w360
              shift-left: w366 -> [w384]
              n157 = Bundle By Name(cluster=w379, "Update Offset Actions"=w374, "Offset Type"=w378, "Coordinate Space"=w377, "Cartesian Type"=w376, "Tag"=w375) -> (w380:T12)
              n158 = Enqueue Element(queue=w383, element=w380, error in (no error)=w384) -> (queue out=w382:refnum<queue>, error out=w381:errorcluster)  [unwired: 1 in, 1 out]
            }
          }
          frame Error {
            n159 = call <vilib>:"Clear Errors.vi"("error in (no error)"=w386) -> ("error out"=w385:errorcluster)  [unwired: 6 in]
          }
        }
        n160 = event-data("Discard?"=TRUE) -> ()  [unwired: 4 in, 1 out]
      }
      event "Cancel": Value Change {
        n161 = event-data() -> ()  [unwired: 2 out]
        n162 = local read "Coordinate Space"() -> (w393:T7)
        n163 = local read "Offset Type"() -> (w394:T8)
        n164 = local read "Cartesian Type"() -> (w392:bool)
        n165 = local read item#-1() -> (w390)
        n166 = Index Array(index=w390) -> (array=w391:string[], element=w389)
        n167 = Bundle By Name(cluster=w396, "Update Offset Actions"=Update_Offset_Actions."Exit" ("notification"), "Offset Type"=w394, "Coordinate Space"=w393, "Cartesian Type"=w392, "Tag"=w389) -> (w395:T12)
        n168 = Enqueue Element(queue=w403, element=w395, error in (no error)=w400) -> (queue out=w402:refnum<queue>, error out=w401:errorcluster)  [unwired: 1 in, 1 out]
        n169 = local read "Default Data"() -> (w398:dbl[][])
        n170 = local read "Default Transactions"() -> (w399:T3[])
        n171 = call "Batch Dataset Store.vi"("Data"=w398, "Transactions"=w399) -> ()  [unwired: 9 in, 1 out]
      }
      event Application Instance Close; Panel Close {
        n172 = event-data() -> ()  [unwired: 2 out]
        n173 = local read "Coordinate Space"() -> (w410:T7)
        n174 = local read "Cartesian Type"() -> (w409:bool)
        n175 = local read "Offset Type"() -> (w411:T8)
        n176 = local read item#-1() -> (w406)
        n177 = Index Array(index=w406) -> (array=w408:string[], element=w407)
        n178 = Bundle By Name(cluster=w413, "Update Offset Actions"=Update_Offset_Actions."Exit" ("notification"), "Offset Type"=w411, "Coordinate Space"=w410, "Cartesian Type"=w409, "Tag"=w407) -> (w414:T12)
        n179 = local read "Default Data"() -> (w415:dbl[][])
        n180 = Enqueue Element(queue=w420, element=w414, error in (no error)=w417) -> (queue out=w419:refnum<queue>, error out=w418:errorcluster)  [unwired: 1 in, 1 out]
        n181 = local read "Default Transactions"() -> (w416:T3[])
        n182 = call "Batch Dataset Store.vi"("Data"=w415, "Transactions"=w416) -> ()  [unwired: 9 in, 1 out]
      }
      event "Execute": Value Change {
        w426 = T13[] [enum."Calculate Cartesian Offsets", enum."Update Table", enum."Has Been Modified"] items=["Update Table", "Calculate Cartesian Offsets", "Redo Headers", "Has Been Modified", "Exit"]
        n183 = event-data() -> ()  [unwired: 2 out]
        n184 = local read "Offset Widget Actions"() -> (w432:T9)
        n185 = Index Array() -> (array=w436:string[], element=w431, index=w425:i32)
        n186 = case shown="\"Calculate External Sensor Offsets\"" w432 {
          selector: w432 -> [w455 w471 _]
          tunnel: w441 -> [w463 w478 _]
          tunnel: [w462 w477 dbl[][] []] -> w440
          tunnel: [w461 w476 w486] -> w438
          tunnel: w431 -> [_ _ w487]
          tunnel: w422 -> [_ w470 _]
          frame "Calculate Displacement Offsets", Default {
            n187 = local read "Number Of Samples"() -> (w456:i32)
            n188 = call "Offset Widget Actions 2 Transactions.vi"("Number of LBCBs"=w463, "Offset Widget Actions"=w455) -> ("Transactions"=w461:T3[])  [unwired: 9 in]
            n189 = Initialize Array(0.0 ("element"), 2 ("dimension size"), 6 ("dimension size")) -> (w457:dbl[][])
            n190 = for {
              N: w456 -> [_]
              shift-right: [w467] -> w464
              shift-left: w457 -> [w469]
              tunnel: w461 -> [w466]
              n191 = local read "Sample Interval\n(milliseconds)"() -> (w468:dbl)
              n192 = call "Batch Dataset Retrieval.vi"("Transactions"=w466) -> ("Data"=w465:dbl[][])  [unwired: 9 in, 1 out]
              n193 = Add(x=w465, y=w469) -> (x+y=w467:dbl[][])
              n194 = Wait Until Next ms Multiple(millisecond multiple=w468) -> ()  [unwired: 1 out]
            }
            n195 = Divide(x=w464, y=w456) -> (x/y=w462:dbl[][])
          }
          frame "Calculate External Sensor Offsets" {
            n196 = local read "Number Of Samples"() -> (w472:i32)
            n197 = call "Offset Widget Actions 2 Transactions.vi"("Number of LBCBs"=w478, "Offset Widget Actions"=w471) -> ("Transactions"=w476:T3[])  [unwired: 9 in]
            n198 = Initialize Array(0.0 ("element"), 2 ("dimension size"), w470) -> (w473:dbl[][])
            n199 = for {
              N: w472 -> [_]
              shift-right: [w481] -> w479
              shift-left: w473 -> [w483]
              tunnel: w476 -> [_]
              n200 = local read "Sample Interval\n(milliseconds)"() -> (w482:dbl)
              n201 = call "Batch Dataset Retrieval.vi"() -> ("Data"=w480:dbl[][])  [unwired: 9 in, 1 out]
              n202 = Add(x=w480, y=w483) -> (x+y=w481:dbl[][])
              n203 = Wait Until Next ms Multiple(millisecond multiple=w482) -> ()  [unwired: 1 out]
            }
            n204 = Divide(x=w479, y=w472) -> (x/y=w477:dbl[][])
          }
          frame "Calculate Displacement Command Offsets" {
            n205 = call "Offsets.vi"("DAO Actions"=DAO_Actions."Get") -> ("Labels"=w488:string[])  [unwired: 8 in, 2 out]
            n206 = for {
              tunnel: w488 -> [w496] mode=indexing
              tunnel: w487 -> [w495]
              shift-right: [w491] -> w486
              shift-left: T3[] [] -> [w490]
              n207 = call "Label 2 Dataset Transaction Id.vi"("Label"=w496) -> ("Dataset Trans Id"=w492:T3)  [unwired: 10 in]
              n208 = Unbundle By Name(w492) -> ("Tag"=w493:string)
              n209 = Equal?(x=w493, y=w495) -> (x = y?=w494:bool)
              n210 = case shown="True" w494 {
                tunnel: w492 -> [_ w500]
                tunnel: [w497 w499] -> w491
                tunnel: w490 -> [w497 w498]
                frame False {
                }
                frame True {
                  n211 = Build Array (concatenate)(w498, w500) -> (w499:T3[])
                }
              }
            }
          }
        }
        n212 = case shown="\"Delete Force Offsets\"" w432 {
          tunnel: w438 -> [w503 w507 w512 w524]
          tunnel: w431 -> [w501 w504 w508 _]
          tunnel: [w503 w506 w512 T3[] [] ("Transactions")] -> w437
          tunnel: w436 -> [_ _ w511 w519]
          tunnel: [w502 w505 w510 w515] -> w433
          tunnel: [w502 w505 w509 w514] -> w435
          tunnel: w425 -> [_ _ _ w518]
          tunnel: [w501 w504 w508 w516] -> w423
          frame "Calculate Displacement Offsets", Default {
          }
          frame "Calculate Force Offsets" {
          }
          frame "Calculate External Sensor Offsets" {
          }
          frame "Calculate Displacement Command Offsets" {
            n213 = Decrement(x=w518) -> (x-1=w522:dbl)
            n214 = for {
              tunnel: w524 -> [w527] mode=indexing
              n215 = call "Offsets.vi"("Dataset Trans Id"=w527, "DAO Actions"=DAO_Actions_with_Remove."Remove") -> ()  [unwired: 7 in, 3 out]
            }
            n216 = Delete From Array(array=w519, length=1, index=w518) -> (array with subset deleted=w513)  [unwired: 1 out]
            n217 = Less Than 0?(x=w522) -> (x < 0?=w523:bool)
            n218 = Select(t=0, s=w523, f=w522) -> (s? t:f=w520:i32)
            n219 = Index Array(array=w513, index=w520) -> (element=w516)
            n220 = local write item#-1(w520) -> ()
          }
        }
        n221 = local read "Coordinate Space"() -> (w429:T7)
        n222 = local read "Cartesian Type"() -> (w427:bool)
        n223 = local read "Offset Type"() -> (w428:T8)
        n224 = for {
          tunnel: w437 -> [w531] mode=indexing
          tunnel: w440 -> [w530] mode=indexing
          shift-right: [w528] -> w439
          shift-left: w435 -> [w529]
          n225 = call "Offsets.vi"("error in (no error)"=w529, "Dataset Trans Id"=w531, "Data In"=w530, "DAO Actions"=DAO_Actions."Set") -> ("error out"=w528:errorcluster)  [unwired: 5 in, 2 out]
        }
        n226 = for {
          tunnel: w430 -> [w449]
          tunnel: w426 -> [w448] mode=indexing
          tunnel: w429 -> [w447]
          tunnel: w428 -> [w446]
          tunnel: w427 -> [w445]
          shift-right: [w452] -> w442
          shift-left: w444 -> [w454]
          shift-right: [w453] -> w443
          shift-left: w439 -> [w451]
          tunnel: w423 -> [_]
          n227 = Bundle By Name(cluster=w449, "Update Offset Actions"=w448, "Offset Type"=w446, "Coordinate Space"=w447, "Cartesian Type"=w445) -> (w450:T12)
          n228 = Enqueue Element(queue=w454, element=w450, error in (no error)=w451) -> (queue out=w452:refnum<queue>, error out=w453:errorcluster)  [unwired: 1 in, 1 out]
        }
      }
      event "Table 0", "Table 1", "Table 2", "Table 3", "Table 4", "Table 5": Value Change {
        w540 = T13[] [enum."Calculate Cartesian Offsets", enum."Update Table", enum."Has Been Modified"] items=["Update Table", "Calculate Cartesian Offsets", "Redo Headers", "Has Been Modified", "Exit"]
        n229 = event-data() -> ("CtlRef"=w554:refnum<vi>, "OldVal"=w550:T2, "NewVal"=w549:T2)  [unwired: 1 out]
        n230 = local read item#-1() -> (w535)
        n231 = local read "Coordinate Space"() -> (w539:T7)
        n232 = Search 1D Array(1D array=w551, element=w554) -> (index of element=w552:i32)  [unwired: 1 in]
        n233 = local read "Offset Type"() -> (w537:T8)
        n234 = Index Array(index=w535) -> (array=w545:string[], element=w534)
        n235 = case shown="\"Forces\", Default" w537 {
          tunnel: w553 -> [w567 w601]
          tunnel: [w566 w600] -> w544
          tunnel: w552 -> [w571 w603]
          tunnel: w551 -> [_ w604]
          tunnel: w550 -> [_ w602]
          tunnel: w539 -> [w576 w599]
          tunnel: w549 -> [w575 w596]
          tunnel: w548 -> [w570 w597]
          tunnel: w547 -> [w569 w598]
          tunnel: w546 -> [w568 _]
          tunnel: w534 -> [_ w595]
          frame "Displacements" {
            n236 = Unbundle By Name(w575) -> ("Table Data 1"=w574:dbl[][])
            n237 = Index Array(array=w574, index (col)=0 ("disabled index (col)")) -> (element=w572:dbl[])  [unwired: 1 in]
            n238 = case shown="True" w576 {
              tunnel: w572 -> [w582 w590]
              tunnel: w571 -> [w580 w593]
              tunnel: w570 -> [_ w588]
              tunnel: w569 -> [w581 w587]
              tunnel: w568 -> [w579 _]
              tunnel: w567 -> [w584 w586]
              tunnel: [w583 w585] -> w566
              frame False {
                n239 = call "Table Number 2 Dataset Source.vi"("Rigid Connection"=w579, "Table Number"=w580, "Number of\nLBCBs"=w581) -> ("Dataset Source"=w578:T4, "IsCommand"=w577:bool)  [unwired: 1 in, 1 out]
                n240 = call "Manual Cartesian Displacement Offset.vi"("error in"=w584, "Cartesian Displacements"=w582, "Dataset Source"=w578, "Is Command"=w577) -> ("error out"=w583:errorcluster)  [unwired: 7 in]
              }
              frame True {
                n241 = call "Displacement Table Number 2 Dataset Id.vi"("Table Number"=w593, "Number of\nLBCBs"=w587) -> ("Dataset Source"=w592:T4, "Dataset Type"=w591:T5)  [unwired: 2 in]
                n242 = Bundle By Name(cluster=w588, "Dataset Type"=w591, "Dataset Source"=w592) -> (w589:T3)
                n243 = call "Offsets.vi"("error in (no error)"=w586, "Dataset Trans Id"=w589, "Data In"=w590, "DAO Actions"=DAO_Actions_with_Remove."Set") -> ("error out"=w585:errorcluster)  [unwired: 5 in, 2 out]
              }
            }
          }
          frame "Forces", Default {
            n244 = case shown="True" w599 {
              tunnel: w604 -> [w611 _]
              tunnel: w603 -> [w610 w618]
              tunnel: w602 -> [w608 _]
              tunnel: w601 -> [w607 w619]
              tunnel: [w606 w620] -> w600
              tunnel: w598 -> [_ _]
              tunnel: w597 -> [_ w617]
              tunnel: w596 -> [_ w616]
              tunnel: w595 -> [_ w612]
              frame False {
                n245 = Index Array(array=w611, index=w610) -> (element=w609:refnum<vi>)
                n246 = property class="Clust (strict)"(reference=w609, error in=w607, "Value"=w608) -> (error out=w606:errorcluster)  [unwired: 1 out]
                n247 = One Button Dialog(message="Manual changes not implemented") -> ()  [unwired: 1 in, 1 out]
              }
              frame True {
                n248 = Unbundle By Name(w616) -> ("Table Data 1"=w615:dbl[][])
                n249 = call "Force Table Number 2 Dataset Id.vi"("Table Number"=w618) -> ("Dataset Source"=w623:T4, "Dataset Type"=w622:T5)  [unwired: 3 in]
                n250 = Index Array(array=w615, index (col)=0 ("disabled index (col)")) -> (element=w613:dbl[])  [unwired: 1 in]
                n251 = Bundle By Name(cluster=w617, "Dataset Type"=w622, "Dataset Source"=w623, "Tag"=w612) -> (w621:T3)
                n252 = call "Offsets.vi"("error in (no error)"=w619, "Dataset Trans Id"=w621, "Data In"=w613, "DAO Actions"=DAO_Actions_with_Remove."Set") -> ("error out"=w620:errorcluster)  [unwired: 5 in, 2 out]
              }
            }
          }
        }
        n253 = local read "Cartesian Type"() -> (w536:bool)
        n254 = for {
          tunnel: w538 -> [w560]
          tunnel: w540 -> [w559] mode=indexing
          tunnel: w536 -> [w556]
          tunnel: w537 -> [w558]
          tunnel: w539 -> [w555]
          tunnel: w534 -> [w557]
          shift-right: [w563] -> w542
          shift-left: w541 -> [w565]
          shift-right: [w564] -> w543
          shift-left: w544 -> [w562]
          n255 = Bundle By Name(cluster=w560, "Update Offset Actions"=w559, "Offset Type"=w558, "Coordinate Space"=w555, "Cartesian Type"=w556, "Tag"=w557) -> (w561:T12)
          n256 = Enqueue Element(queue=w565, element=w561, error in (no error)=w562) -> (queue out=w563:refnum<queue>, error out=w564:errorcluster)  [unwired: 1 in, 1 out]
        }
      }
      event Timeout {
        n257 = event-data() -> ()  [unwired: 4 out]
        n258 = local write "Execute"(FALSE ("Calculate")) -> ()
        n259 = local read "Offset Type"() -> (w627:T8)
        n260 = local read item#-1() -> (w628)
        n261 = local read "Coordinate Space"() -> (w626:T7)
        n262 = local read "Cartesian Type"() -> (w625:bool)
        n263 = Index Array(index=w628) -> (array=w629:string[], element=w637)
        n264 = Bundle By Name(cluster=w630, "Update Offset Actions"=Update_Offset_Actions."Update Table" ("element"), "Offset Type"=w627, "Coordinate Space"=w626, "Cartesian Type"=w625, "Tag"=w637) -> (w631:T12)
        n265 = Enqueue Element(queue=w635, element=w631, error in (no error)=w632) -> (queue out=w634:refnum<queue>, error out=w633:errorcluster)  [unwired: 1 in, 1 out]
      }
    }
  }
  "error out" <- w25
  n266 = Compound Arithmetic op=AND(w24, w23) -> (w22:bool)
  n267 = flat-sequence {
    tunnel: w22 -> [w645]
    frame #0 {
      n268 = Not(x=w645) -> (.not. x?=w644:bool)
      n269 = local write "Cancel"(w644) -> ()
      n270 = control-ref of="This VI"() -> (w641:refnum<vi>)
      n271 = local write "Ok"(w644) -> ()
      n272 = property class="VI"(reference=w641) -> ("Front Panel.Open"=w640:bool)  [unwired: 1 in, 2 out]
      n273 = case shown="True" w640 {
        tunnel: w641 -> [_ w646]
        frame False {
        }
        frame True {
          n274 = invoke class="VI" method="FP.Close"(reference=w646) -> ()  [unwired: 2 in, 3 out]
        }
      }
      n275 = call "NoArgumentsLauncher.vi"("Application"=NoPanelAppTypes."Offsets", "Application Launcher Actions"=Launcher_Actions."Stop") -> ()  [unwired: 1 in, 9 out]
    }
  }
